vi "ATS_SetExternalTrigger.vi"(10 "ExtTrigControl":T1, 11 "DeviceIn":i32) -> (0 "Return Code":u32, 3 "DeviceOut":i32)   [LabVIEW 2014]
doc: "_____AlazarTech, Scope_____\n\nConfigure the external trigger circuitry.\n\n- Coupling\n- External Trigger Range"
uses:
  ATS_ctl/ExtTrigger.ctl
  ATS_ctl/Coupling.ctl
  ATS_ctl/ExtTrigRange.ctl
  ATS_ctl/ATS_Global_Ctrl.ctl
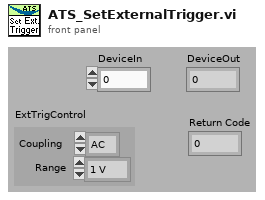
[diagram p1: front panel]
types:
  T1 = typedef "ExtTrigger.ctl" = cluster{"Coupling":T2, "Range":T3}
  T2 = typedef "Coupling.ctl" = enum16{"AC", "DC"}
  T3 = typedef "ExtTrigRange.ctl" = enum16{"1 V", "5 V", "TTL"}
  T4 = typedef "ATS_Global_Ctrl.ctl" = enum16{"Init_Device", "Clear_ALL", "Set", "Get"}
  T5 = typedef "ATS_Set_Value.ctl" = cluster{"Clock (s)":dbl, "RangeA (v)":dbl, "RangeB (v)":dbl, "Ranges (v)":dbl[]}
  T6 = typedef "ATS_Global_4Ch.ctl" = cluster{"Record":T7, "Clock":T8, "Inputs":T12, "Trigger":T17}
  T7 = typedef "Record.ctl" = cluster{"Count":u32, "Presize":u32, "Length":u32}
  T8 = typedef "Clock.ctl" = cluster{"ClckSource":T9, "ClckRate":T10, "ClckEdge":T11, "Decimation":u32}
  T9 = typedef "ClockSource.ctl" = enum16{"Internal", "External", "Medium Ext.", "Slow Ext.", "Ext. AC", "Ext. DC", "Ext. (PLL)"}
  T10 = typedef "ClockRate.ctl" = u32
  T11 = typedef "ClockEdge.ctl" = u16
  T12 = typedef "ATS_InputArray.ctl" = T13[]
  T13 = typedef "InputCtrl.ctl" = cluster{"Coupling":T2, "Range":T14, "Impedance":T15, "Bandwidth":T16}
  T14 = typedef "Range.ctl" = u32
  T15 = typedef "Impedance.ctl" = enum16{"1M ohms", "50 ohms"}
  T16 = typedef "Bandwidth.ctl" = enum16{"Full Bandwidth", "Reduce Bandwidth"}
  T17 = typedef "ATS_Trigger_4Ch.ctl" = cluster{"TrigOperation":T18, "Timeout (s)":dbl, "Trig. Delay":u32, "Engine X":T19, "Engine Y":T19, "ExtTrigControl":T1}
  T18 = typedef "TriggerOperation.ctl" = enum16{"Only X", "Only Y", "X or Y", "X and Y", "X xor Y", "X and not Y", "not X and Y"}
  T19 = typedef "ATS_TriggerEngine_4Ch.ctl" = cluster{"Source":T20, "Slope":enum32{"Positive", "Negative"}, "Level":u32}
  T20 = typedef "ATS_TriggerSource_4Ch.ctl" = enum32{"Chan_A", "Chan_B", "External", "Disable", "Chan_C", "Chan_D"}
  T21 = typedef "Device_Info.ctl" = cluster{"Handle":u32, "Board":string, "CPLD":string, "MemorySize":u32, "SampleSize":u8, "ID":i32, "High_Memory":bool, "Chan/Board":u8}
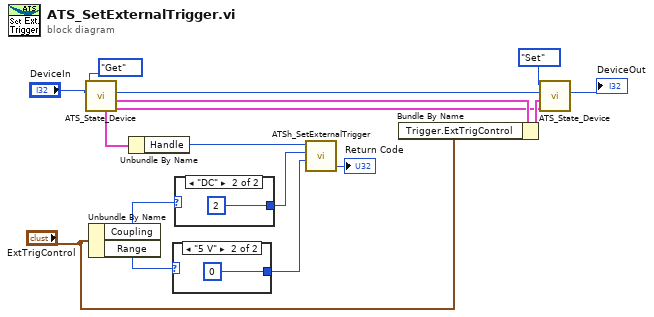
[diagram p0: block diagram]
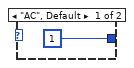
[diagram p2: hidden frame]
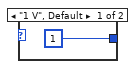
[diagram p3: hidden frame]
diagram:
  n1 = call "ATS_State_Device.vi"("DeviceIn"="DeviceIn", "ATS_GBL_Ctrl"=ATS_Global_Ctrl."Get") -> ("Ref_Out"=w5:T5, "SetupOut"=w7:T6, "DeviceOut"=w12:i32, "DevInfo_Out"=w6:T21)  [unwired: 4 in, 2 out]
  n2 = Unbundle By Name("ExtTrigControl") -> ("Coupling"=w16:T2, "Range"=w15:T3)
  n3 = Unbundle By Name(w6) -> ("Handle"=w3:u32)
  n4 = case shown="\"5 V\"" w15 {
    tunnel: [u32 1 ("Channel") u32 0 ("Channel")] -> w1
    frame "1 V", Default {
    }
    frame "5 V" {
    }
  }
  n5 = case shown="\"DC\"" w16 {
    tunnel: [u32 1 ("Channel") u32 2 ("Channel")] -> w2
    frame "AC", Default {
    }
    frame "DC" {
    }
  }
  n6 = call "ATSh_SetExternalTrigger.vi"("Range"=w1, "Coupling"=w2, "Handle"=w3) -> ("Return"=→"Return Code":u32)  [unwired: 7 in, 1 out]
  n7 = Bundle By Name(cluster=w7, "Trigger.ExtTrigControl"="ExtTrigControl") -> (w9:T6)
  n8 = call "ATS_State_Device.vi"("Ref_In"=w5, "SetupIn"=w9, "DeviceIn"=w12, "ATS_GBL_Ctrl"=ATS_Global_Ctrl."Set") -> ("DeviceOut"=→"DeviceOut":i32)  [unwired: 2 in, 5 out]
